vi "Lab Panel V5.28.vi"() -> ()   [LabVIEW 2013] (continued)
                    n2201 = Multiply(x=w3854, y=w3848) -> (x*y=w3840:dbl)
                    n2202 = local read "SIG LAB02-1"() -> (w3847:T2)
                    n2203 = local read "SIG LAB02-2"() -> (w3843:T2)
                    n2204 = Bundle By Name(cluster=w3847, "AMPS"=w3846, "VOLTS"=w3845, "PF"=w3844) -> (w3839:T2)
                    n2205 = Bundle By Name(cluster=w3843, "AMPS"=w3842, "VOLTS"=w3841, "PF"=w3840) -> (w3838:T2)
                    n2206 = global write "Global display 1.vi" "SIG LAB02-1"(w3839) -> ()
                    n2207 = local write "SIG LAB02-2"(w3838) -> ()
                    n2208 = global write "Global display 1.vi" "SIG LAB02-2"(w3838) -> ()
                    n2209 = local write "SIG LAB02-1"(w3839) -> ()
                  }
                  frame #4 {
                    n2210 = Unbundle By Name(w3891) -> ("OFF amps"=w3887:dbl, "VOLTS"=w3886:dbl, "PF"=w3885:dbl, "OFF amps"=w3884:dbl, "VOLTS"=w3883:dbl, "PF"=w3882:dbl)
                    n2211 = case shown="True" w3890 {
                      tunnel: [w3892 w3893] -> w3888
                      tunnel: w3889 -> [_ w3893]
                      frame False {
                        n2212 = local read "CAL LAB03"() -> (w3892:T14)
                      }
                      frame True {
                      }
                    }
                    n2213 = Unbundle By Name(w3888) -> ("1  (A) cal"=w3881:dbl, "1 (V) cal"=w3880:dbl, "1 (PF) cal"=w3879:dbl, "2 (A) cal"=w3878:dbl, "2 (V) cal"=w3877:dbl, "2 (PF) cal"=w3876:dbl)  [unwired: 4 out]
                    n2214 = Multiply(x=w3887, y=w3881) -> (x*y=w3874:dbl)
                    n2215 = Multiply(x=w3886, y=w3880) -> (x*y=w3868:dbl)
                    n2216 = Multiply(x=w3885, y=w3879) -> (x*y=w3873:dbl)
                    n2217 = Multiply(x=w3884, y=w3878) -> (x*y=w3871:dbl)
                    n2218 = Multiply(x=w3883, y=w3877) -> (x*y=w3870:dbl)
                    n2219 = Multiply(x=w3882, y=w3876) -> (x*y=w3869:dbl)
                    n2220 = local read "SIG LAB03-1"() -> (w3875:T2)
                    n2221 = local read "SIG LAB03-2"() -> (w3872:T2)
                    n2222 = Bundle By Name(cluster=w3875, "AMPS"=w3874, "VOLTS"=w3868, "PF"=w3873) -> (w3867:T2)
                    n2223 = Bundle By Name(cluster=w3872, "AMPS"=w3871, "VOLTS"=w3870, "PF"=w3869) -> (w3866:T2)
                    n2224 = global write "Global display 1.vi" "SIG LAB03-1"(w3867) -> ()
                    n2225 = global write "Global display 1.vi" "SIG LAB03-2"(w3866) -> ()
                    n2226 = local write "SIG LAB03-2"(w3866) -> ()
                    n2227 = local write "SIG LAB03-1"(w3867) -> ()
                  }
                  frame #5 {
                    n2228 = case shown="False" w3918 {
                      tunnel: [w3920 w3921] -> w3916
                      tunnel: w3917 -> [_ w3921]
                      frame False {
                        n2229 = local read "CAL LAB04"() -> (w3920:T14)
                      }
                      frame True {
                      }
                    }
                    n2230 = Unbundle By Name(w3919) -> ("OFF amps"=w3915:dbl, "VOLTS"=w3914:dbl, "PF"=w3913:dbl, "OFF amps"=w3912:dbl, "VOLTS"=w3911:dbl, "PF"=w3910:dbl)
                    n2231 = Unbundle By Name(w3916) -> ("1  (A) cal"=w3909:dbl, "1 (V) cal"=w3908:dbl, "1 (PF) cal"=w3907:dbl, "2 (A) cal"=w3906:dbl, "2 (V) cal"=w3905:dbl, "2 (PF) cal"=w3904:dbl)  [unwired: 4 out]
                    n2232 = Multiply(x=w3915, y=w3909) -> (x*y=w3902:dbl)
                    n2233 = Multiply(x=w3914, y=w3908) -> (x*y=w3901:dbl)
                    n2234 = Multiply(x=w3913, y=w3907) -> (x*y=w3900:dbl)
                    n2235 = Multiply(x=w3912, y=w3906) -> (x*y=w3898:dbl)
                    n2236 = Multiply(x=w3911, y=w3905) -> (x*y=w3897:dbl)
                    n2237 = Multiply(x=w3910, y=w3904) -> (x*y=w3896:dbl)
                    n2238 = local read "SIG LAB04-1"() -> (w3903:T2)
                    n2239 = local read "SIG LAB04-2"() -> (w3899:T2)
                    n2240 = Bundle By Name(cluster=w3903, "AMPS"=w3902, "VOLTS"=w3901, "PF"=w3900) -> (w3895:T2)
                    n2241 = Bundle By Name(cluster=w3899, "AMPS"=w3898, "VOLTS"=w3897, "PF"=w3896) -> (w3894:T2)
                    n2242 = global write "Global display 1.vi" "SIG LAB04-2"(w3894) -> ()
                    n2243 = global write "Global display 1.vi" "SIG LAB04-1"(w3895) -> ()
                    n2244 = local write "SIG LAB04-2"(w3894) -> ()
                    n2245 = local write "SIG LAB04-1"(w3895) -> ()
                  }
                  frame #6 {
                    n2246 = Unbundle By Name(w3947) -> ("OFF amps"=w3943:dbl, "VOLTS"=w3924:dbl, "PF"=w3942:dbl, "OFF amps"=w3941:dbl, "VOLTS"=w3940:dbl, "PF"=w3939:dbl)
                    n2247 = case shown="False" w3946 {
                      tunnel: [w3948 w3949] -> w3944
                      tunnel: w3945 -> [_ w3949]
                      frame False {
                        n2248 = local read "CAL LAB05"() -> (w3948:T14)
                      }
                      frame True {
                      }
                    }
                    n2249 = Unbundle By Name(w3944) -> ("1  (A) cal"=w3938:dbl, "1 (V) cal"=w3937:dbl, "1 (PF) cal"=w3936:dbl, "2 (A) cal"=w3935:dbl, "2 (V) cal"=w3934:dbl, "2 (PF) cal"=w3933:dbl)  [unwired: 4 out]
                    n2250 = Multiply(x=w3943, y=w3938) -> (x*y=w3931:dbl)
                    n2251 = Multiply(x=w3924, y=w3937) -> (x*y=w3930:dbl)
                    n2252 = Multiply(x=w3942, y=w3936) -> (x*y=w3929:dbl)
                    n2253 = Multiply(x=w3941, y=w3935) -> (x*y=w3927:dbl)
                    n2254 = Multiply(x=w3940, y=w3934) -> (x*y=w3926:dbl)
                    n2255 = Multiply(x=w3939, y=w3933) -> (x*y=w3925:dbl)
                    n2256 = local read "SIG LAB05-1"() -> (w3932:T2)
                    n2257 = local read "SIG LAB05-2"() -> (w3928:T2)
                    n2258 = Bundle By Name(cluster=w3932, "AMPS"=w3931, "VOLTS"=w3930, "PF"=w3929) -> (w3923:T2)
                    n2259 = Bundle By Name(cluster=w3928, "AMPS"=w3927, "VOLTS"=w3926, "PF"=w3925) -> (w3922:T2)
                    n2260 = global write "Global display 1.vi" "SIG LAB05-1"(w3923) -> ()
                    n2261 = global write "Global display 1.vi" "SIG LAB05-2"(w3922) -> ()
                    n2262 = local write "SIG LAB05-2"(w3922) -> ()
                    n2263 = local write "SIG LAB05-1"(w3923) -> ()
                  }
                  frame #7 {
                    n2264 = case shown="False" w3950 {
                      tunnel: w3952 -> [w3957 _]
                      tunnel: w3951 -> [w3956 _]
                      frame False {
                        # "update ambient referance temperature"
                        n2265 = case shown="True" w3957 {
                          tunnel: [w3959 100.0] -> w3958
                          frame False {
                            n2266 = local read "TEMP REF cal"() -> (w3959:dbl)
                          }
                          frame True {
                          }
                        }
                        n2267 = disable-structure shown="Disabled" {
                          frame Disabled {
                            n2268 = local read "Temp read loop"() -> ()  [unwired: 1 out]
                          }
                          frame Enabled {
                          }
                        }
                        n2269 = Multiply(x=w3958, y=w3956) -> (x*y=w3955:dbl)
                        n2270 = Subtract(x=w3955, y=272) -> (x-y=w3953:dbl)
                        "Amb Tp" <- w3953
                        n2271 = local write "Ref deg C"(w3953) -> ()
                        "deg C (volts)" <- w3956
                      }
                      frame True {
                      }
                    }
                  }
                }
              }
            }
          }
          frame #14 {
            # "save test data to file during testing"
            n2272 = local read "on loops"() -> (w3980:dbl)
            n2273 = Get Date/Time In Seconds() -> (seconds since 1Jan1904=w3961:timestamp)
            "File Time Stamp" <- w3961
            n2274 = local read "jig cycle"() -> (w3977:dbl)
            n2275 = Format Date/Time String(time format string (%c)="%H:%M%:%S", seconds (now)=w3961) -> (date/time string=w3965:string)  [unwired: 1 in]
            n2276 = Add(x=w3980, y=4) -> (x+y=w3978:dbl)
            n2277 = Build Array(w3965) -> (w3964:string[])
            n2278 = Equal?(x=w3977, y=3) -> (x = y?=w3963:bool)
            n2279 = Equal?(x=w3977, y=w3978) -> (x = y?=w3962:bool)
            n2280 = stacked-sequence {
              tunnel: w3976 -> [w3986 _ _ _ _ _ _ _ _ _]
              tunnel: w3975 -> [_ w4062 _ _ _ _ _ _ _ _]
              tunnel: w3974 -> [_ _ w4142 _ _ _ _ _ _ _]
              tunnel: w3973 -> [_ _ _ w4222 _ _ _ _ _ _]
              tunnel: w3972 -> [_ _ _ _ w4302 _ _ _ _ _]
              tunnel: w3971 -> [_ _ _ _ _ w4382 _ _ _ _]
              tunnel: w3970 -> [_ _ _ _ _ _ w4462 _ _ _]
              tunnel: w3969 -> [_ _ _ _ _ _ _ w4542 _ _]
              tunnel: w3968 -> [_ _ _ _ _ _ _ _ w4622 _]
              tunnel: w3967 -> [_ _ _ _ _ _ _ _ _ w4702]
              tunnel: w3964 -> [w3985 w4066 w4146 w4226 w4306 w4386 w4466 w4546 w4626 w4706]
              tunnel: w3963 -> [w3984 w4065 w4145 w4225 w4305 w4385 w4465 w4545 w4625 w4705]
              tunnel: w3962 -> [w3983 w4064 w4144 w4224 w4304 w4384 w4464 w4544 w4624 w4704]
              tunnel: w3961 -> [w3982 w4063 w4143 w4223 w4303 w4383 w4463 w4543 w4623 w4703]
              frame #0 {
                n2281 = case shown="True" w3986 {
                  tunnel: w3985 -> [_ w3991]
                  tunnel: w3984 -> [_ w3990]
                  tunnel: w3983 -> [_ w3988]
                  tunnel: w3982 -> [_ w3987]
                  frame False {
                  }
                  frame True {
                    n2282 = local read "DISP LAB01-1"() -> (w3992:T4)
                    n2283 = local read "SIG LAB01-1"() -> (w3993:T2)
                    n2284 = local read "ON L01-1"() -> (w3989:cluster{"amps":dbl, "volts":dbl, "pf":dbl})
                    n2285 = Unbundle(w3993) -> ("AMPS"=w3999:dbl, "VOLTS"=w3997:dbl, "PF"=w3996:dbl, "Tmp Live"=w3995:dbl, "Tmp Neut"=w3998:dbl)
                    n2286 = Unbundle(w3992) -> ("CYCLE"=w3994:dbl)  [unwired: 2 out]
                    n2287 = stacked-sequence {
                      tunnel: w3999 -> [w4003 w4022]
                      tunnel: w3998 -> [_ w4021]
                      tunnel: w3997 -> [w4002 w4020]
                      tunnel: w3996 -> [w4001 w4019]
                      tunnel: w3995 -> [_ w4018]
                      tunnel: w3994 -> [_ w4017]
                      tunnel: w3991 -> [_ w4016]
                      tunnel: w3990 -> [w4004 _]
                      tunnel: w3989 -> [w4000 w4014]
                      tunnel: w3988 -> [_ w4015]
                      tunnel: w3987 -> [_ w4010]
                      frame #0 {
                        n2288 = case shown="True" w4004 {
                          tunnel: w4003 -> [_ w4009]
                          tunnel: w4002 -> [_ w4008]
                          tunnel: w4001 -> [_ w4007]
                          tunnel: w4000 -> [_ w4005]
                          frame False {
                          }
                          frame True {
                            n2289 = Bundle(cluster=w4005, "amps"=w4009, "volts"=w4008, "pf"=w4007) -> (w4006:cluster{"amps":dbl, "volts":dbl, "pf":dbl})
                            n2290 = local write "ON L01-1"(w4006) -> ()
                          }
                        }
                      }
                      frame #1 {
                        n2291 = Unbundle(w4014) -> ("amps"=w4013:dbl, "volts"=w4012:dbl, "pf"=w4011:dbl)
                        n2292 = case shown="True" w4015 {
                          tunnel: w4022 -> [_ w4023]
                          tunnel: w4021 -> [_ w4061]
                          tunnel: w4020 -> [_ _]
                          tunnel: w4019 -> [_ _]
                          tunnel: w4018 -> [_ w4060]
                          tunnel: w4017 -> [_ w4059]
                          tunnel: w4016 -> [_ w4027]
                          tunnel: w4013 -> [_ w4024]
                          tunnel: w4012 -> [_ w4056]
                          tunnel: w4011 -> [_ w4055]
                          tunnel: w4010 -> [_ w4025]
                          frame False {
                          }
                          frame True {
                            n2293 = local read "TDMS LAB01-1"() -> (w4058:refnum<k34>)
                            n2294 = Build Array(w4056) -> (w4052:dbl[])
                            n2295 = Build Array(w4055) -> (w4051:dbl[])
                            n2296 = Build Array(w4060) -> (w4050:dbl[])
                            n2297 = Build Array(w4061) -> (w4049:dbl[])
                            n2298 = Build Array(w4024) -> (w4054:dbl[])
                            n2299 = Build Array(w4023) -> (w4053:dbl[])
                            n2300 = Build Array(w4059) -> (w4048:dbl[])
                            n2301 = Build Array("AMPS ON", "AMPS OFF", "VOLTS", "PF", "TEMP Live", "TEMP Neut", "CYCLE") -> (w4032:string[])
                            n2302 = Bundle By Name("Y"=w4054, "t0"=w4025) -> (w4047:waveform(dbl))  [unwired: 1 in]
                            n2303 = Bundle By Name("Y"=w4053, "t0"=w4025) -> (w4046:waveform(dbl))  [unwired: 1 in]
                            n2304 = Bundle By Name("Y"=w4052, "t0"=w4025) -> (w4045:waveform(dbl))  [unwired: 1 in]
                            n2305 = Bundle By Name("Y"=w4051, "t0"=w4025) -> (w4044:waveform(dbl))  [unwired: 1 in]
                            n2306 = Bundle By Name("Y"=w4050, "t0"=w4025) -> (w4043:waveform(dbl))  [unwired: 1 in]
                            n2307 = Bundle By Name("Y"=w4049, "t0"=w4025) -> (w4042:waveform(dbl))  [unwired: 1 in]
                            n2308 = Bundle By Name("Y"=w4048, "t0"=w4025) -> (w4041:waveform(dbl))  [unwired: 1 in]
                            n2309 = Build Array(w4047, w4046, w4045, w4044, w4043, w4042, w4041) -> (w4040:waveform(dbl)[])
                            n2310 = TDMS Write(0:w4058, 5:"TEST VALUES", 7:w4032, 9:w4040) -> (4:w4031:refnum<k34>, 6:w4030:string, 15:w4029:errorcluster)  [unwired: 2 in, 1 out]
                            n2311 = TDMS Write(0:w4031, 5:w4030, 7:"TIME", 9:w4027, 11:w4029) -> (15:w4026:errorcluster)  [unwired: 1 in, 3 out]
                            n2312 = local write "data file error"(w4026) -> ()
                          }
                        }
                      }
                    }
                  }
                }
              }
              frame #1 {
                n2313 = case shown="True" w4062 {
                  tunnel: w4066 -> [_ w4071]
                  tunnel: w4065 -> [_ w4070]
                  tunnel: w4064 -> [_ w4068]
                  tunnel: w4063 -> [_ w4067]
                  frame False {
                  }
                  frame True {
                    n2314 = local read "DISP LAB01-2"() -> (w4072:T4)
                    n2315 = local read "SIG LAB01-2"() -> (w4073:T2)
                    n2316 = local read "ON L01-2"() -> (w4069:cluster{"amps":dbl, "volts":dbl, "pf":dbl})
                    n2317 = Unbundle(w4073) -> ("AMPS"=w4079:dbl, "VOLTS"=w4077:dbl, "PF"=w4076:dbl, "Tmp Live"=w4075:dbl, "Tmp Neut"=w4078:dbl)
                    n2318 = Unbundle(w4072) -> ("CYCLE"=w4074:dbl)  [unwired: 2 out]
                    n2319 = stacked-sequence {
                      tunnel: w4079 -> [w4083 w4102]
                      tunnel: w4078 -> [_ w4101]
                      tunnel: w4077 -> [w4082 w4100]
                      tunnel: w4076 -> [w4081 w4099]
                      tunnel: w4075 -> [_ w4098]
                      tunnel: w4074 -> [_ w4097]
                      tunnel: w4071 -> [_ w4096]
                      tunnel: w4070 -> [w4084 _]
                      tunnel: w4069 -> [w4080 w4094]
                      tunnel: w4068 -> [_ w4095]
                      tunnel: w4067 -> [_ w4090]
                      frame #0 {
                        n2320 = case shown="True" w4084 {
                          tunnel: w4083 -> [_ w4089]
                          tunnel: w4082 -> [_ w4088]
                          tunnel: w4081 -> [_ w4087]
                          tunnel: w4080 -> [_ w4085]
                          frame False {
                          }
                          frame True {
                            n2321 = Bundle(cluster=w4085, "amps"=w4089, "volts"=w4088, "pf"=w4087) -> (w4086:cluster{"amps":dbl, "volts":dbl, "pf":dbl})
                            n2322 = local write "ON L01-2"(w4086) -> ()
                          }
                        }
                      }
                      frame #1 {
                        n2323 = Unbundle(w4094) -> ("amps"=w4093:dbl, "volts"=w4092:dbl, "pf"=w4091:dbl)
                        n2324 = case shown="True" w4095 {
                          tunnel: w4102 -> [_ w4134]
                          tunnel: w4101 -> [_ w4141]
                          tunnel: w4100 -> [_ _]
                          tunnel: w4099 -> [_ _]
                          tunnel: w4098 -> [_ w4140]
                          tunnel: w4097 -> [_ w4139]
                          tunnel: w4096 -> [_ w4104]
                          tunnel: w4093 -> [_ w4136]
                          tunnel: w4092 -> [_ w4135]
                          tunnel: w4091 -> [_ w4133]
                          tunnel: w4090 -> [_ w4125]
                          frame False {
                          }
                          frame True {
                            n2325 = local read "TDMS LAB01-2"() -> (w4138:refnum<k34>)
                            n2326 = Build Array(w4135) -> (w4130:dbl[])
                            n2327 = Build Array(w4133) -> (w4129:dbl[])
                            n2328 = Build Array(w4140) -> (w4128:dbl[])
                            n2329 = Build Array(w4141) -> (w4127:dbl[])
                            n2330 = Build Array(w4136) -> (w4132:dbl[])
                            n2331 = Build Array(w4134) -> (w4131:dbl[])
                            n2332 = Build Array(w4139) -> (w4126:dbl[])
                            n2333 = Build Array("AMPS ON", "AMPS OFF", "VOLTS", "PF", "TEMP Live", "TEMP Neut", "CYCLE") -> (w4109:string[])
                            n2334 = Bundle By Name("Y"=w4132, "t0"=w4125) -> (w4124:waveform(dbl))  [unwired: 1 in]
                            n2335 = Bundle By Name("Y"=w4131, "t0"=w4125) -> (w4123:waveform(dbl))  [unwired: 1 in]
                            n2336 = Bundle By Name("Y"=w4130, "t0"=w4125) -> (w4122:waveform(dbl))  [unwired: 1 in]
                            n2337 = Bundle By Name("Y"=w4129, "t0"=w4125) -> (w4121:waveform(dbl))  [unwired: 1 in]
                            n2338 = Bundle By Name("Y"=w4128, "t0"=w4125) -> (w4120:waveform(dbl))  [unwired: 1 in]
                            n2339 = Bundle By Name("Y"=w4127, "t0"=w4125) -> (w4119:waveform(dbl))  [unwired: 1 in]
                            n2340 = Bundle By Name("Y"=w4126, "t0"=w4125) -> (w4118:waveform(dbl))  [unwired: 1 in]
                            n2341 = Build Array(w4124, w4123, w4122, w4121, w4120, w4119, w4118) -> (w4117:waveform(dbl)[])
                            n2342 = TDMS Write(0:w4138, 5:"TEST VALUES", 7:w4109, 9:w4117) -> (4:w4108:refnum<k34>, 6:w4107:string, 15:w4106:errorcluster)  [unwired: 2 in, 1 out]
                            n2343 = TDMS Write(0:w4108, 5:w4107, 7:"TIME", 9:w4104, 11:w4106) -> (15:w4103:errorcluster)  [unwired: 1 in, 3 out]
                            n2344 = local write "data file error"(w4103) -> ()
                          }
                        }
                      }
                    }
                  }
                }
              }
              frame #2 {
                n2345 = case shown="True" w4142 {
                  tunnel: w4146 -> [_ w4151]
                  tunnel: w4145 -> [_ w4150]
                  tunnel: w4144 -> [_ w4148]
                  tunnel: w4143 -> [_ w4147]
                  frame False {
                  }
                  frame True {
                    n2346 = local read "DISP LAB02-1"() -> (w4152:T4)
                    n2347 = local read "SIG LAB02-1"() -> (w4153:T2)
                    n2348 = local read "ON L02-1"() -> (w4149:cluster{"amps":dbl, "volts":dbl, "pf":dbl})
                    n2349 = Unbundle(w4153) -> ("AMPS"=w4159:dbl, "VOLTS"=w4157:dbl, "PF"=w4156:dbl, "Tmp Live"=w4155:dbl, "Tmp Neut"=w4158:dbl)
                    n2350 = Unbundle(w4152) -> ("CYCLE"=w4154:dbl)  [unwired: 2 out]
                    n2351 = stacked-sequence {
                      tunnel: w4159 -> [w4163 w4182]
                      tunnel: w4158 -> [_ w4181]
                      tunnel: w4157 -> [w4162 w4180]
                      tunnel: w4156 -> [w4161 w4179]
                      tunnel: w4155 -> [_ w4178]
                      tunnel: w4154 -> [_ w4177]
                      tunnel: w4151 -> [_ w4176]
                      tunnel: w4150 -> [w4164 _]
                      tunnel: w4149 -> [w4160 w4174]
                      tunnel: w4148 -> [_ w4175]
                      tunnel: w4147 -> [_ w4170]
                      frame #0 {
                        n2352 = case shown="True" w4164 {
                          tunnel: w4163 -> [_ w4169]
                          tunnel: w4162 -> [_ w4168]
                          tunnel: w4161 -> [_ w4167]
                          tunnel: w4160 -> [_ w4165]
                          frame False {
                          }
                          frame True {
                            n2353 = Bundle(cluster=w4165, "amps"=w4169, "volts"=w4168, "pf"=w4167) -> (w4166:cluster{"amps":dbl, "volts":dbl, "pf":dbl})
                            n2354 = local write "ON L02-1"(w4166) -> ()
                          }
                        }
                      }
                      frame #1 {
                        n2355 = Unbundle(w4174) -> ("amps"=w4173:dbl, "volts"=w4172:dbl, "pf"=w4171:dbl)
                        n2356 = case shown="True" w4175 {
                          tunnel: w4182 -> [_ w4214]
                          tunnel: w4181 -> [_ w4221]
                          tunnel: w4180 -> [_ _]
                          tunnel: w4179 -> [_ _]
                          tunnel: w4178 -> [_ w4220]
                          tunnel: w4177 -> [_ w4219]
                          tunnel: w4176 -> [_ w4184]
                          tunnel: w4173 -> [_ w4216]
                          tunnel: w4172 -> [_ w4215]
                          tunnel: w4171 -> [_ w4213]
                          tunnel: w4170 -> [_ w4205]
                          frame False {
                          }
                          frame True {
                            n2357 = local read "TDMS LAB02-1"() -> (w4218:refnum<k34>)
                            n2358 = Build Array(w4215) -> (w4210:dbl[])
                            n2359 = Build Array(w4213) -> (w4209:dbl[])
                            n2360 = Build Array(w4220) -> (w4208:dbl[])
                            n2361 = Build Array(w4221) -> (w4207:dbl[])
                            n2362 = Build Array(w4216) -> (w4212:dbl[])
                            n2363 = Build Array(w4214) -> (w4211:dbl[])
                            n2364 = Build Array(w4219) -> (w4206:dbl[])
                            n2365 = Build Array("AMPS ON", "AMPS OFF", "VOLTS", "PF", "TEMP Live", "TEMP Neut", "CYCLE") -> (w4189:string[])
                            n2366 = Bundle By Name("Y"=w4212, "t0"=w4205) -> (w4204:waveform(dbl))  [unwired: 1 in]
                            n2367 = Bundle By Name("Y"=w4211, "t0"=w4205) -> (w4203:waveform(dbl))  [unwired: 1 in]
                            n2368 = Bundle By Name("Y"=w4210, "t0"=w4205) -> (w4202:waveform(dbl))  [unwired: 1 in]
                            n2369 = Bundle By Name("Y"=w4209, "t0"=w4205) -> (w4201:waveform(dbl))  [unwired: 1 in]
                            n2370 = Bundle By Name("Y"=w4208, "t0"=w4205) -> (w4200:waveform(dbl))  [unwired: 1 in]
                            n2371 = Bundle By Name("Y"=w4207, "t0"=w4205) -> (w4199:waveform(dbl))  [unwired: 1 in]
                            n2372 = Bundle By Name("Y"=w4206, "t0"=w4205) -> (w4198:waveform(dbl))  [unwired: 1 in]
                            n2373 = Build Array(w4204, w4203, w4202, w4201, w4200, w4199, w4198) -> (w4197:waveform(dbl)[])
                            n2374 = TDMS Write(0:w4218, 5:"TEST VALUES", 7:w4189, 9:w4197) -> (4:w4188:refnum<k34>, 6:w4187:string, 15:w4186:errorcluster)  [unwired: 2 in, 1 out]
                            n2375 = TDMS Write(0:w4188, 5:w4187, 7:"TIME", 9:w4184, 11:w4186) -> (15:w4183:errorcluster)  [unwired: 1 in, 3 out]
                            n2376 = local write "data file error"(w4183) -> ()
                          }
                        }
                      }
                    }
                  }
                }
              }
              frame #3 {
                n2377 = case shown="True" w4222 {
                  tunnel: w4226 -> [_ w4231]
                  tunnel: w4225 -> [_ w4230]
                  tunnel: w4224 -> [_ w4228]
                  tunnel: w4223 -> [_ w4227]
                  frame False {
                  }
                  frame True {
                    n2378 = local read "DISP LAB02-2"() -> (w4232:T4)
                    n2379 = local read "SIG LAB02-2"() -> (w4233:T2)
                    n2380 = local read "ON L02-2"() -> (w4229:cluster{"amps":dbl, "volts":dbl, "pf":dbl})
                    n2381 = Unbundle(w4233) -> ("AMPS"=w4239:dbl, "VOLTS"=w4237:dbl, "PF"=w4236:dbl, "Tmp Live"=w4235:dbl, "Tmp Neut"=w4238:dbl)
                    n2382 = Unbundle(w4232) -> ("CYCLE"=w4234:dbl)  [unwired: 2 out]
                    n2383 = stacked-sequence {
                      tunnel: w4239 -> [w4243 w4262]
                      tunnel: w4238 -> [_ w4261]
                      tunnel: w4237 -> [w4242 w4260]
                      tunnel: w4236 -> [w4241 w4259]
                      tunnel: w4235 -> [_ w4258]
                      tunnel: w4234 -> [_ w4257]
                      tunnel: w4231 -> [_ w4256]
                      tunnel: w4230 -> [w4244 _]
                      tunnel: w4229 -> [w4240 w4254]
                      tunnel: w4228 -> [_ w4255]
                      tunnel: w4227 -> [_ w4250]
                      frame #0 {
                        n2384 = case shown="True" w4244 {
                          tunnel: w4243 -> [_ w4249]
                          tunnel: w4242 -> [_ w4248]
                          tunnel: w4241 -> [_ w4247]
                          tunnel: w4240 -> [_ w4245]
                          frame False {
                          }
                          frame True {
                            n2385 = Bundle(cluster=w4245, "amps"=w4249, "volts"=w4248, "pf"=w4247) -> (w4246:cluster{"amps":dbl, "volts":dbl, "pf":dbl})
                            n2386 = local write "ON L02-2"(w4246) -> ()
                          }
                        }
                      }
                      frame #1 {
                        n2387 = Unbundle(w4254) -> ("amps"=w4253:dbl, "volts"=w4252:dbl, "pf"=w4251:dbl)
                        n2388 = case shown="True" w4255 {
                          tunnel: w4262 -> [_ w4294]
                          tunnel: w4261 -> [_ w4301]
                          tunnel: w4260 -> [_ _]
                          tunnel: w4259 -> [_ _]
                          tunnel: w4258 -> [_ w4300]
                          tunnel: w4257 -> [_ w4299]
                          tunnel: w4256 -> [_ w4264]
                          tunnel: w4253 -> [_ w4296]
                          tunnel: w4252 -> [_ w4295]
                          tunnel: w4251 -> [_ w4293]
                          tunnel: w4250 -> [_ w4285]
                          frame False {
                          }
                          frame True {
                            n2389 = local read "TDMS LAB02-2"() -> (w4298:refnum<k34>)
                            n2390 = Build Array(w4295) -> (w4290:dbl[])
                            n2391 = Build Array(w4293) -> (w4289:dbl[])
                            n2392 = Build Array(w4300) -> (w4288:dbl[])
                            n2393 = Build Array(w4301) -> (w4287:dbl[])
                            n2394 = Build Array(w4296) -> (w4292:dbl[])
                            n2395 = Build Array(w4294) -> (w4291:dbl[])
                            n2396 = Build Array(w4299) -> (w4286:dbl[])
                            n2397 = Build Array("AMPS ON", "AMPS OFF", "VOLTS", "PF", "TEMP Live", "TEMP Neut", "CYCLE") -> (w4269:string[])
                            n2398 = Bundle By Name("Y"=w4292, "t0"=w4285) -> (w4284:waveform(dbl))  [unwired: 1 in]
                            n2399 = Bundle By Name("Y"=w4291, "t0"=w4285) -> (w4283:waveform(dbl))  [unwired: 1 in]
                            n2400 = Bundle By Name("Y"=w4290, "t0"=w4285) -> (w4282:waveform(dbl))  [unwired: 1 in]
                            n2401 = Bundle By Name("Y"=w4289, "t0"=w4285) -> (w4281:waveform(dbl))  [unwired: 1 in]
                            n2402 = Bundle By Name("Y"=w4288, "t0"=w4285) -> (w4280:waveform(dbl))  [unwired: 1 in]
                            n2403 = Bundle By Name("Y"=w4287, "t0"=w4285) -> (w4279:waveform(dbl))  [unwired: 1 in]
                            n2404 = Bundle By Name("Y"=w4286, "t0"=w4285) -> (w4278:waveform(dbl))  [unwired: 1 in]
                            n2405 = Build Array(w4284, w4283, w4282, w4281, w4280, w4279, w4278) -> (w4277:waveform(dbl)[])
                            n2406 = TDMS Write(0:w4298, 5:"TEST VALUES", 7:w4269, 9:w4277) -> (4:w4268:refnum<k34>, 6:w4267:string, 15:w4266:errorcluster)  [unwired: 2 in, 1 out]
                            n2407 = TDMS Write(0:w4268, 5:w4267, 7:"TIME", 9:w4264, 11:w4266) -> (15:w4263:errorcluster)  [unwired: 1 in, 3 out]
                            n2408 = local write "data file error"(w4263) -> ()
                          }
                        }
                      }
                    }
                  }
                }
              }
              frame #4 {
                n2409 = case shown="True" w4302 {
                  tunnel: w4306 -> [_ w4311]
                  tunnel: w4305 -> [_ w4310]
                  tunnel: w4304 -> [_ w4308]
                  tunnel: w4303 -> [_ w4307]
                  frame False {
                  }
                  frame True {
                    n2410 = local read "DISP LAB03-1"() -> (w4312:T4)
                    n2411 = local read "SIG LAB03-1"() -> (w4313:T2)
                    n2412 = local read "ON L03-1"() -> (w4309:cluster{"amps":dbl, "volts":dbl, "pf":dbl})
                    n2413 = Unbundle(w4313) -> ("AMPS"=w4319:dbl, "VOLTS"=w4317:dbl, "PF"=w4316:dbl, "Tmp Live"=w4315:dbl, "Tmp Neut"=w4318:dbl)
                    n2414 = Unbundle(w4312) -> ("CYCLE"=w4314:dbl)  [unwired: 2 out]
                    n2415 = stacked-sequence {
                      tunnel: w4319 -> [w4323 w4342]
                      tunnel: w4318 -> [_ w4341]
                      tunnel: w4317 -> [w4322 w4340]
                      tunnel: w4316 -> [w4321 w4339]
                      tunnel: w4315 -> [_ w4338]
                      tunnel: w4314 -> [_ w4337]
                      tunnel: w4311 -> [_ w4336]
                      tunnel: w4310 -> [w4324 _]
                      tunnel: w4309 -> [w4320 w4334]
                      tunnel: w4308 -> [_ w4335]
                      tunnel: w4307 -> [_ w4330]
                      frame #0 {
                        n2416 = case shown="True" w4324 {
                          tunnel: w4323 -> [_ w4329]
                          tunnel: w4322 -> [_ w4328]
                          tunnel: w4321 -> [_ w4327]
                          tunnel: w4320 -> [_ w4325]
                          frame False {
                          }
                          frame True {
                            n2417 = Bundle(cluster=w4325, "amps"=w4329, "volts"=w4328, "pf"=w4327) -> (w4326:cluster{"amps":dbl, "volts":dbl, "pf":dbl})
                            n2418 = local write "ON L03-1"(w4326) -> ()
                          }
                        }
                      }
                      frame #1 {
                        n2419 = Unbundle(w4334) -> ("amps"=w4333:dbl, "volts"=w4332:dbl, "pf"=w4331:dbl)
                        n2420 = case shown="True" w4335 {
                          tunnel: w4342 -> [_ w4374]
                          tunnel: w4341 -> [_ w4381]
                          tunnel: w4340 -> [_ _]
                          tunnel: w4339 -> [_ _]
                          tunnel: w4338 -> [_ w4380]
                          tunnel: w4337 -> [_ w4379]
                          tunnel: w4336 -> [_ w4344]
                          tunnel: w4333 -> [_ w4376]
                          tunnel: w4332 -> [_ w4375]
                          tunnel: w4331 -> [_ w4373]
                          tunnel: w4330 -> [_ w4365]
                          frame False {
                          }
                          frame True {
                            n2421 = local read "TDMS LAB03-1"() -> (w4378:refnum<k34>)
                            n2422 = Build Array(w4375) -> (w4370:dbl[])
                            n2423 = Build Array(w4373) -> (w4369:dbl[])
                            n2424 = Build Array(w4380) -> (w4368:dbl[])
                            n2425 = Build Array(w4381) -> (w4367:dbl[])
                            n2426 = Build Array(w4376) -> (w4372:dbl[])
                            n2427 = Build Array(w4374) -> (w4371:dbl[])
                            n2428 = Build Array(w4379) -> (w4366:dbl[])
                            n2429 = Build Array("AMPS ON", "AMPS OFF", "VOLTS", "PF", "TEMP Live", "TEMP Neut", "CYCLE") -> (w4349:string[])
                            n2430 = Bundle By Name("Y"=w4372, "t0"=w4365) -> (w4364:waveform(dbl))  [unwired: 1 in]
                            n2431 = Bundle By Name("Y"=w4371, "t0"=w4365) -> (w4363:waveform(dbl))  [unwired: 1 in]
                            n2432 = Bundle By Name("Y"=w4370, "t0"=w4365) -> (w4362:waveform(dbl))  [unwired: 1 in]
                            n2433 = Bundle By Name("Y"=w4369, "t0"=w4365) -> (w4361:waveform(dbl))  [unwired: 1 in]
                            n2434 = Bundle By Name("Y"=w4368, "t0"=w4365) -> (w4360:waveform(dbl))  [unwired: 1 in]
                            n2435 = Bundle By Name("Y"=w4367, "t0"=w4365) -> (w4359:waveform(dbl))  [unwired: 1 in]
                            n2436 = Bundle By Name("Y"=w4366, "t0"=w4365) -> (w4358:waveform(dbl))  [unwired: 1 in]
                            n2437 = Build Array(w4364, w4363, w4362, w4361, w4360, w4359, w4358) -> (w4357:waveform(dbl)[])
                            n2438 = TDMS Write(0:w4378, 5:"TEST VALUES", 7:w4349, 9:w4357) -> (4:w4348:refnum<k34>, 6:w4347:string, 15:w4346:errorcluster)  [unwired: 2 in, 1 out]
                            n2439 = TDMS Write(0:w4348, 5:w4347, 7:"TIME", 9:w4344, 11:w4346) -> (15:w4343:errorcluster)  [unwired: 1 in, 3 out]
                            n2440 = local write "data file error"(w4343) -> ()
                          }
                        }
                      }
                    }
                  }
                }
              }
              frame #5 {
                n2441 = case shown="True" w4382 {
                  tunnel: w4386 -> [_ w4391]
                  tunnel: w4385 -> [_ w4390]
                  tunnel: w4384 -> [_ w4388]
                  tunnel: w4383 -> [_ w4387]
                  frame False {
                  }
                  frame True {
                    n2442 = local read "DISP LAB03-2"() -> (w4392:T4)
                    n2443 = local read "SIG LAB03-2"() -> (w4393:T2)
                    n2444 = local read "ON L03-2"() -> (w4389:cluster{"amps":dbl, "volts":dbl, "pf":dbl})
                    n2445 = Unbundle(w4393) -> ("AMPS"=w4399:dbl, "VOLTS"=w4397:dbl, "PF"=w4396:dbl, "Tmp Live"=w4395:dbl, "Tmp Neut"=w4398:dbl)
                    n2446 = Unbundle(w4392) -> ("CYCLE"=w4394:dbl)  [unwired: 2 out]
                    n2447 = stacked-sequence {
                      tunnel: w4399 -> [w4403 w4422]
                      tunnel: w4398 -> [_ w4421]
                      tunnel: w4397 -> [w4402 w4420]
                      tunnel: w4396 -> [w4401 w4419]
                      tunnel: w4395 -> [_ w4418]
                      tunnel: w4394 -> [_ w4417]
                      tunnel: w4391 -> [_ w4416]
                      tunnel: w4390 -> [w4404 _]
                      tunnel: w4389 -> [w4400 w4414]
                      tunnel: w4388 -> [_ w4415]
                      tunnel: w4387 -> [_ w4410]
                      frame #0 {
                        n2448 = case shown="True" w4404 {
                          tunnel: w4403 -> [_ w4409]
                          tunnel: w4402 -> [_ w4408]
                          tunnel: w4401 -> [_ w4407]
                          tunnel: w4400 -> [_ w4405]
                          frame False {
                          }
                          frame True {
                            n2449 = Bundle(cluster=w4405, "amps"=w4409, "volts"=w4408, "pf"=w4407) -> (w4406:cluster{"amps":dbl, "volts":dbl, "pf":dbl})
                            n2450 = local write "ON L03-2"(w4406) -> ()
                          }
                        }
                      }
                      frame #1 {
                        n2451 = Unbundle(w4414) -> ("amps"=w4413:dbl, "volts"=w4412:dbl, "pf"=w4411:dbl)
                        n2452 = case shown="True" w4415 {
                          tunnel: w4422 -> [_ w4454]
                          tunnel: w4421 -> [_ w4461]
                          tunnel: w4420 -> [_ _]
                          tunnel: w4419 -> [_ _]
                          tunnel: w4418 -> [_ w4460]
                          tunnel: w4417 -> [_ w4459]
                          tunnel: w4416 -> [_ w4424]
                          tunnel: w4413 -> [_ w4456]
                          tunnel: w4412 -> [_ w4455]
                          tunnel: w4411 -> [_ w4453]
                          tunnel: w4410 -> [_ w4445]
                          frame False {
                          }
                          frame True {
                            n2453 = local read "TDMS LAB03-2"() -> (w4458:refnum<k34>)
                            n2454 = Build Array(w4455) -> (w4450:dbl[])
                            n2455 = Build Array(w4453) -> (w4449:dbl[])
                            n2456 = Build Array(w4460) -> (w4448:dbl[])
                            n2457 = Build Array(w4461) -> (w4447:dbl[])
                            n2458 = Build Array(w4456) -> (w4452:dbl[])
                            n2459 = Build Array(w4454) -> (w4451:dbl[])
                            n2460 = Build Array(w4459) -> (w4446:dbl[])
                            n2461 = Build Array("AMPS ON", "AMPS OFF", "VOLTS", "PF", "TEMP Live", "TEMP Neut", "CYCLE") -> (w4429:string[])
                            n2462 = Bundle By Name("Y"=w4452, "t0"=w4445) -> (w4444:waveform(dbl))  [unwired: 1 in]
                            n2463 = Bundle By Name("Y"=w4451, "t0"=w4445) -> (w4443:waveform(dbl))  [unwired: 1 in]
                            n2464 = Bundle By Name("Y"=w4450, "t0"=w4445) -> (w4442:waveform(dbl))  [unwired: 1 in]
                            n2465 = Bundle By Name("Y"=w4449, "t0"=w4445) -> (w4441:waveform(dbl))  [unwired: 1 in]
                            n2466 = Bundle By Name("Y"=w4448, "t0"=w4445) -> (w4440:waveform(dbl))  [unwired: 1 in]
                            n2467 = Bundle By Name("Y"=w4447, "t0"=w4445) -> (w4439:waveform(dbl))  [unwired: 1 in]
                            n2468 = Bundle By Name("Y"=w4446, "t0"=w4445) -> (w4438:waveform(dbl))  [unwired: 1 in]
                            n2469 = Build Array(w4444, w4443, w4442, w4441, w4440, w4439, w4438) -> (w4437:waveform(dbl)[])
                            n2470 = TDMS Write(0:w4458, 5:"TEST VALUES", 7:w4429, 9:w4437) -> (4:w4428:refnum<k34>, 6:w4427:string, 15:w4426:errorcluster)  [unwired: 2 in, 1 out]
                            n2471 = TDMS Write(0:w4428, 5:w4427, 7:"TIME", 9:w4424, 11:w4426) -> (15:w4423:errorcluster)  [unwired: 1 in, 3 out]
                            n2472 = local write "data file error"(w4423) -> ()
                          }
                        }
                      }
                    }
                  }
                }
              }
              frame #6 {
                n2473 = case shown="True" w4462 {
                  tunnel: w4466 -> [_ w4471]
                  tunnel: w4465 -> [_ w4470]
                  tunnel: w4464 -> [_ w4468]
                  tunnel: w4463 -> [_ w4467]
                  frame False {
                  }
                  frame True {
                    n2474 = local read "DISP LAB04-1"() -> (w4472:T4)
                    n2475 = local read "SIG LAB04-1"() -> (w4473:T2)
                    n2476 = local read "ON L04-1"() -> (w4469:cluster{"amps":dbl, "volts":dbl, "pf":dbl})
                    n2477 = Unbundle(w4473) -> ("AMPS"=w4479:dbl, "VOLTS"=w4477:dbl, "PF"=w4476:dbl, "Tmp Live"=w4475:dbl, "Tmp Neut"=w4478:dbl)
                    n2478 = Unbundle(w4472) -> ("CYCLE"=w4474:dbl)  [unwired: 2 out]
                    n2479 = stacked-sequence {
                      tunnel: w4479 -> [w4483 w4502]
                      tunnel: w4478 -> [_ w4501]
                      tunnel: w4477 -> [w4482 w4500]
                      tunnel: w4476 -> [w4481 w4499]
                      tunnel: w4475 -> [_ w4498]
                      tunnel: w4474 -> [_ w4497]
                      tunnel: w4471 -> [_ w4496]
                      tunnel: w4470 -> [w4484 _]
                      tunnel: w4469 -> [w4480 w4494]
                      tunnel: w4468 -> [_ w4495]
                      tunnel: w4467 -> [_ w4490]
                      frame #0 {
                        n2480 = case shown="True" w4484 {
                          tunnel: w4483 -> [_ w4489]
                          tunnel: w4482 -> [_ w4488]
                          tunnel: w4481 -> [_ w4487]
                          tunnel: w4480 -> [_ w4485]
                          frame False {
                          }
                          frame True {
                            n2481 = Bundle(cluster=w4485, "amps"=w4489, "volts"=w4488, "pf"=w4487) -> (w4486:cluster{"amps":dbl, "volts":dbl, "pf":dbl})
                            n2482 = local write "ON L04-1"(w4486) -> ()
                          }
                        }
                      }
                      frame #1 {
                        n2483 = Unbundle(w4494) -> ("amps"=w4493:dbl, "volts"=w4492:dbl, "pf"=w4491:dbl)
                        n2484 = case shown="True" w4495 {
                          tunnel: w4502 -> [_ w4534]
                          tunnel: w4501 -> [_ w4541]
                          tunnel: w4500 -> [_ _]
                          tunnel: w4499 -> [_ _]
                          tunnel: w4498 -> [_ w4540]
                          tunnel: w4497 -> [_ w4539]
                          tunnel: w4496 -> [_ w4504]
                          tunnel: w4493 -> [_ w4536]
                          tunnel: w4492 -> [_ w4535]
                          tunnel: w4491 -> [_ w4533]
                          tunnel: w4490 -> [_ w4525]
                          frame False {
                          }
                          frame True {
                            n2485 = local read "TDMS LAB04-1"() -> (w4538:refnum<k34>)
                            n2486 = Build Array(w4535) -> (w4530:dbl[])
                            n2487 = Build Array(w4533) -> (w4529:dbl[])
                            n2488 = Build Array(w4540) -> (w4528:dbl[])
                            n2489 = Build Array(w4541) -> (w4527:dbl[])
                            n2490 = Build Array(w4536) -> (w4532:dbl[])
                            n2491 = Build Array(w4534) -> (w4531:dbl[])
                            n2492 = Build Array(w4539) -> (w4526:dbl[])
                            n2493 = Build Array("AMPS ON", "AMPS OFF", "VOLTS", "PF", "TEMP Live", "TEMP Neut", "CYCLE") -> (w4509:string[])
                            n2494 = Bundle By Name("Y"=w4532, "t0"=w4525) -> (w4524:waveform(dbl))  [unwired: 1 in]
                            n2495 = Bundle By Name("Y"=w4531, "t0"=w4525) -> (w4523:waveform(dbl))  [unwired: 1 in]
                            n2496 = Bundle By Name("Y"=w4530, "t0"=w4525) -> (w4522:waveform(dbl))  [unwired: 1 in]
                            n2497 = Bundle By Name("Y"=w4529, "t0"=w4525) -> (w4521:waveform(dbl))  [unwired: 1 in]
                            n2498 = Bundle By Name("Y"=w4528, "t0"=w4525) -> (w4520:waveform(dbl))  [unwired: 1 in]
                            n2499 = Bundle By Name("Y"=w4527, "t0"=w4525) -> (w4519:waveform(dbl))  [unwired: 1 in]
                            n2500 = Bundle By Name("Y"=w4526, "t0"=w4525) -> (w4518:waveform(dbl))  [unwired: 1 in]
                            n2501 = Build Array(w4524, w4523, w4522, w4521, w4520, w4519, w4518) -> (w4517:waveform(dbl)[])
                            n2502 = TDMS Write(0:w4538, 5:"TEST VALUES", 7:w4509, 9:w4517) -> (4:w4508:refnum<k34>, 6:w4507:string, 15:w4506:errorcluster)  [unwired: 2 in, 1 out]
                            n2503 = TDMS Write(0:w4508, 5:w4507, 7:"TIME", 9:w4504, 11:w4506) -> (15:w4503:errorcluster)  [unwired: 1 in, 3 out]
                            n2504 = local write "data file error"(w4503) -> ()
                          }
                        }
                      }
                    }
                  }
                }
              }
              frame #7 {
                n2505 = case shown="True" w4542 {
                  tunnel: w4546 -> [_ w4551]
                  tunnel: w4545 -> [_ w4550]
                  tunnel: w4544 -> [_ w4548]
                  tunnel: w4543 -> [_ w4547]
                  frame False {
                  }
                  frame True {
                    n2506 = local read "DISP LAB04-2"() -> (w4552:T4)
                    n2507 = local read "SIG LAB04-2"() -> (w4553:T2)
                    n2508 = local read "ON L04-2"() -> (w4549:cluster{"amps":dbl, "volts":dbl, "pf":dbl})
                    n2509 = Unbundle(w4553) -> ("AMPS"=w4559:dbl, "VOLTS"=w4557:dbl, "PF"=w4556:dbl, "Tmp Live"=w4555:dbl, "Tmp Neut"=w4558:dbl)
                    n2510 = Unbundle(w4552) -> ("CYCLE"=w4554:dbl)  [unwired: 2 out]
                    n2511 = stacked-sequence {
                      tunnel: w4559 -> [w4563 w4582]
                      tunnel: w4558 -> [_ w4581]
                      tunnel: w4557 -> [w4562 w4580]
                      tunnel: w4556 -> [w4561 w4579]
                      tunnel: w4555 -> [_ w4578]
                      tunnel: w4554 -> [_ w4577]
                      tunnel: w4551 -> [_ w4576]
                      tunnel: w4550 -> [w4564 _]
                      tunnel: w4549 -> [w4560 w4574]
                      tunnel: w4548 -> [_ w4575]
                      tunnel: w4547 -> [_ w4570]
                      frame #0 {
                        n2512 = case shown="True" w4564 {
                          tunnel: w4563 -> [_ w4569]
                          tunnel: w4562 -> [_ w4568]
                          tunnel: w4561 -> [_ w4567]
                          tunnel: w4560 -> [_ w4565]
                          frame False {
                          }
                          frame True {
                            n2513 = Bundle(cluster=w4565, "amps"=w4569, "volts"=w4568, "pf"=w4567) -> (w4566:cluster{"amps":dbl, "volts":dbl, "pf":dbl})
                            n2514 = local write "ON L04-2"(w4566) -> ()
                          }
                        }
                      }
                      frame #1 {
                        n2515 = Unbundle(w4574) -> ("amps"=w4573:dbl, "volts"=w4572:dbl, "pf"=w4571:dbl)
                        n2516 = case shown="True" w4575 {
                          tunnel: w4582 -> [_ w4614]
                          tunnel: w4581 -> [_ w4621]
                          tunnel: w4580 -> [_ _]
                          tunnel: w4579 -> [_ _]
                          tunnel: w4578 -> [_ w4620]
                          tunnel: w4577 -> [_ w4619]
                          tunnel: w4576 -> [_ w4584]
                          tunnel: w4573 -> [_ w4616]
                          tunnel: w4572 -> [_ w4615]
                          tunnel: w4571 -> [_ w4613]
                          tunnel: w4570 -> [_ w4605]
                          frame False {
                          }
                          frame True {
                            n2517 = local read "TDMS LAB04-2"() -> (w4618:refnum<k34>)
                            n2518 = Build Array(w4615) -> (w4610:dbl[])
                            n2519 = Build Array(w4613) -> (w4609:dbl[])
                            n2520 = Build Array(w4620) -> (w4608:dbl[])
                            n2521 = Build Array(w4621) -> (w4607:dbl[])
                            n2522 = Build Array(w4616) -> (w4612:dbl[])
                            n2523 = Build Array(w4614) -> (w4611:dbl[])
                            n2524 = Build Array(w4619) -> (w4606:dbl[])
